vi "NF LI56xx dvr sDATA DELete.vi"(8 "error in":errorcluster caption="error in (no error)" {"code" format="%.0x"}, 11 "VISA resource name":refnum<visa-resource-name>) -> (0 "error out":errorcluster {"code" format="%.0x"}, 3 "VISA resource name copy":refnum<visa-resource-name>)   [LabVIEW 2019]
doc: "Clears the specified measurement data buffer."
panel:
  in  "set data buffer":enum16{"BUF1", "BUF2", "BUF3"}(ring)=enum."BUF2"
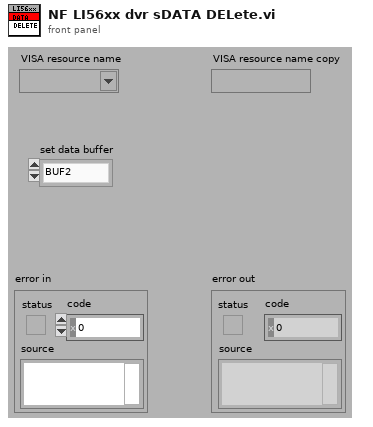
[diagram p1: front panel]
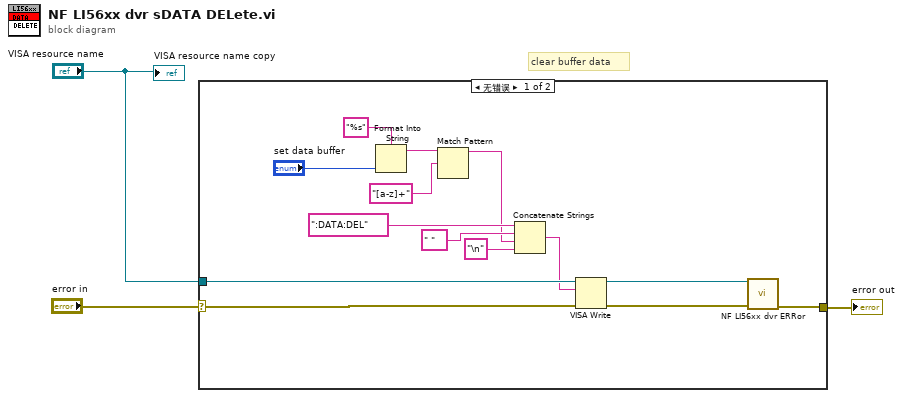
[diagram p0: block diagram]
diagram:
  # "clear buffer data"
  n1 = case shown="无错误" "error in" {
    selector: "error in" -> [w17 w18]
    tunnel: [w13 w18] -> w3
    tunnel: "VISA resource name" -> [w16 _]
    frame No Error {
      n2 = Format Into String(format string="%s", "set data buffer") -> (resulting string=w7:string)  [unwired: 2 in, 1 out]
      n3 = Match Pattern(string=w7, regular expression="[a-z]+") -> (before substring=w4:string)  [unwired: 1 in, 3 out]
      n4 = Concatenate Strings(":DATA:DEL" ("•¶Žš—ñ"), " ", w4, "\n" ("Œ`Ž®•¶Žš—ñ")) -> (w12:string)
      n5 = VISA Write(VISA resource name=w16, write buffer=w12, error in (no error)=w17) -> (VISA resource name out=w15:refnum<visa-resource-name>, error out=w14:errorcluster)  [unwired: 1 out]
      n6 = call "NF LI56xx dvr ERRor.vi"("VISA resource name"=w15, "error in (no error)"=w14) -> ("error out"=w13:errorcluster)  [unwired: 10 in, 3 out]
    }
    frame Error {
    }
  }
  "error out" <- w3
  "VISA resource name copy" <- "VISA resource name"
